vi "DAQmx Create Channel (AI-Voltage-Custom with Excitation).vi"(0 "task in":refnum<k21>, 1 "maximum value":dbl=10.0 format="%0.2f", 2 "minimum value":dbl=-10.0 format="%0.2f", 3 "input terminal configuration":i32(ring)=-1 items=["Default"=-1, "RSE"=10083, "NRSE"=10078, "Differential"=10106, "Pseudodifferential"=12529], 5 "physical channels":tag, 6 "use excitation for scaling":bool, 7 "name to assign":string, 9 "units":i32(ring)=10348 items=["Volts"=10348, "From Custom Scale"=10065], 10 "voltage excitation value":dbl format="%.6f", 11 "error in":errorcluster, 12 "custom scale name":tag, 13 "voltage excitation source":i32(ring)=10200 items=["Internal"=10200, "External"=10167, "None"=10230], 14 "bridge configuration":i32(ring)=10228 items=["Full Bridge"=10182, "Half Bridge"=10187, "Quarter Bridge"=10270, "No Bridge"=10228]) -> (4 "task out":refnum<k21>, 15 "error out":errorcluster)   [LabVIEW 2020]
doc: "Creates channel(s) to measure voltage. Use this instance for custom sensors that require excitation. You can use the excitation to scale the measurement."
uses:
  nilvaiu.dll
panel:
  # "input limits"
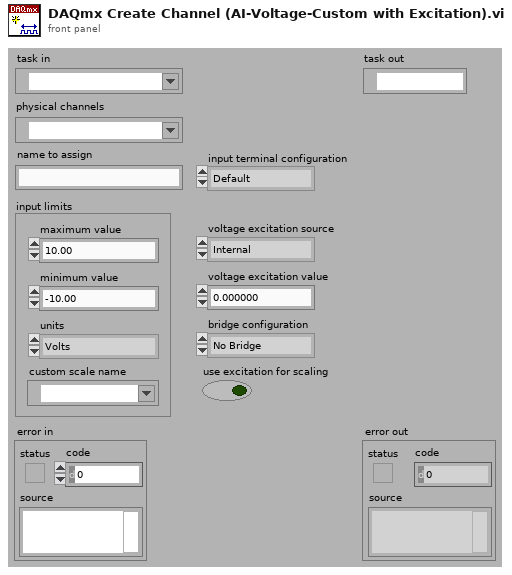
[diagram p1: front panel]
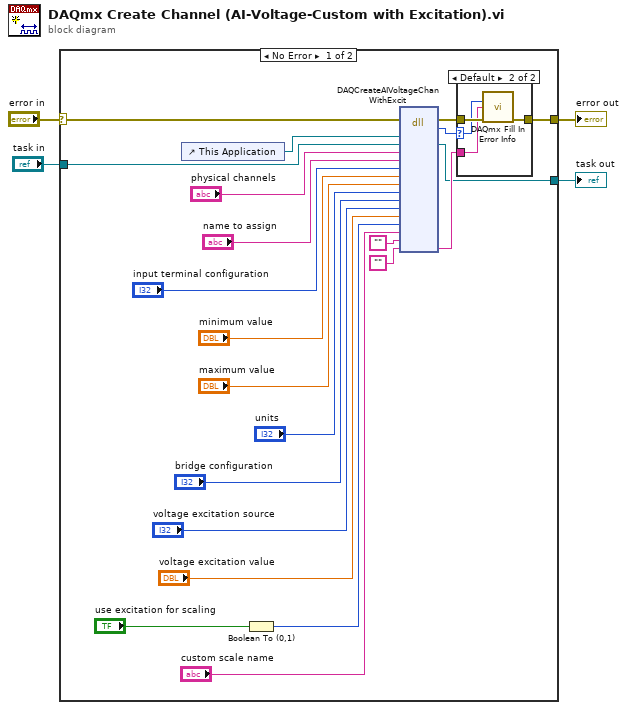
[diagram p0: block diagram]
diagram:
  n1 = case shown="No Error" "error in" {
    selector: "error in" -> [w8 w32]
    tunnel: "task in" -> [w10 w33]
    tunnel: [w9 w33] -> w3
    tunnel: [w7 w32] -> w1
    frame No Error {
      n2 = control-ref of="This Application"() -> (w11:refnum<vi>)
      n3 = Boolean To (0,1)(Boolean="use excitation for scaling") -> (0, 1=w18:i16)
      n4 = dll-call lib="nilvaiu.*" fn="DAQCreateAIVoltageChanWithExcit"(error in=w8, "lvAppRef"=w11, "refObjPtr"=w10, "physicalChannelName"="physical channels", "channelNameIn"="name to assign", "terminalConfig"="input terminal configuration", "minVal"="minimum value", "maxVal"="maximum value", "units"="units", "bridgeConfig"="bridge configuration", "excitSource"="voltage excitation source", "excitVal"="voltage excitation value", "useExcitForScaling"=w18, "customScaleName"="custom scale name", "channelNamesOut"="", "extendedErrorInfo"="") -> (error out=w26:errorcluster, "return type"=w24:i32, "refObjPtr"=w9:refnum<k21>, "extendedErrorInfo"=w22:string)  [unwired: 15 in, 1 out]
      n5 = case shown="Default" w24 {
        selector: w24 -> [_ w29]
        tunnel: w26 -> [w27 w31]
        tunnel: [w27 w30] -> w7
        tunnel: w22 -> [_ w28]
        frame 0 {
        }
        frame Default {
          n6 = call "DAQmx Fill In Error Info.vi"("status code"=w29, "extended error info"=w28, "error in"=w31) -> ("error out"=w30:errorcluster)  [unwired: 1 in, 11 out]
        }
      }
    }
    frame Error {
    }
  }
  "task out" <- w3
  "error out" <- w1
